vi "VIPM_Identify New and Modified Spec Files.vi"(7 "Force Reload?(F)":bool, 8 "error in (no error)":errorcluster, 11 "Spec Files":path[](array[path])) -> (0 "error out":errorcluster, 2 "New or Modified Spec Files":path[](array[path]), 3 "Unchanged Package Array":T1[](array[typedef]))   [LabVIEW 2019]
uses:
  Ctl/Ctl_Package Identifier Cluster.ctl
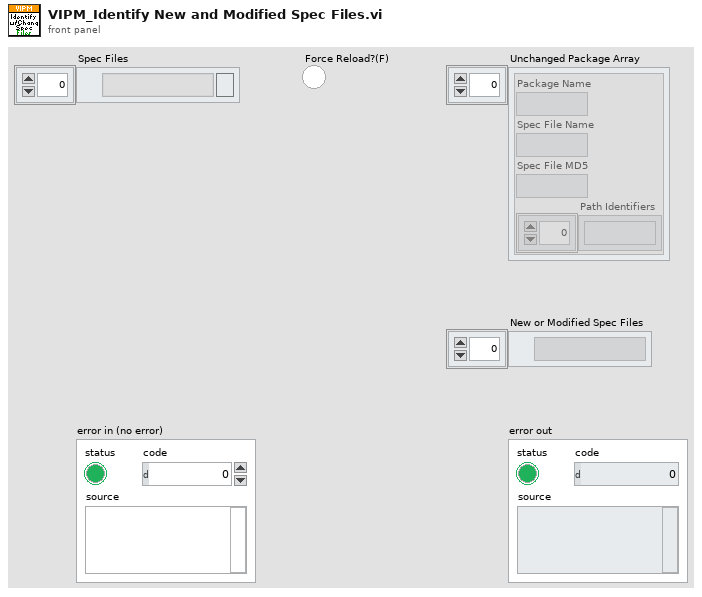
[diagram p1: front panel]
types:
  T1 = typedef "Ctl_Package Identifier Cluster.ctl" = cluster{"Package Name":string, "Spec File Name":string, "Spec File MD5":string, "Path Identifiers":string[]}
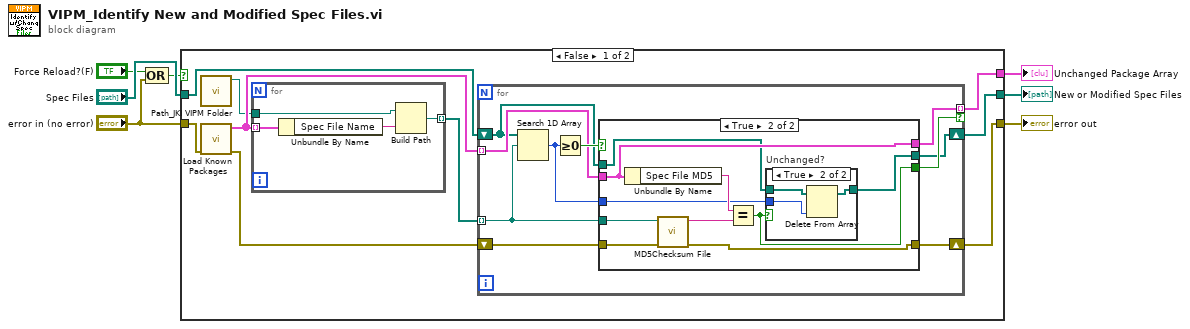
[diagram p0: block diagram]
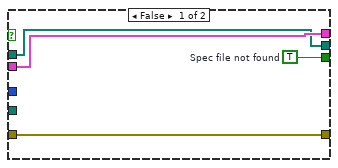
[diagram p2: hidden frame]
diagram:
  n1 = Compound Arithmetic op=OR("Force Reload?(F)", "error in (no error)") -> (w3:bool)
  n2 = case shown="False" w3 {
    tunnel: "Spec Files" -> [w13 w50]
    tunnel: [w12 _] -> w6
    tunnel: [w11 w50] -> w5
    tunnel: [w9 w49] -> w4
    tunnel: "error in (no error)" -> [w8 w49]
    frame False {
      n3 = call "Path_JKI VIPM Folder.vi"() -> ("JKI\\VIPM path"=w14:path)  [unwired: 10 in, 1 out]
      n4 = call "Load Known Packages.vi"("error in (no error)"=w8) -> ("error out"=w10:errorcluster, "Package Array from File"=w16:T1[])  [unwired: 8 in, 1 out]
      n5 = for {
        tunnel: w16 -> [w20] mode=indexing
        tunnel: [w17] -> w15 mode=indexing
        tunnel: w14 -> [w19]
        n6 = Unbundle By Name(w20) -> ("Spec File Name"=w18:string)
        n7 = Build Path(base path=w19, name or relative path=w18) -> (appended path=w17:path)
      }
      n8 = for {
        tunnel: w15 -> [w27] mode=indexing
        tunnel: w16 -> [w26] mode=indexing
        shift-right: [w23] -> w11
        shift-left: w13 -> [w24]
        tunnel: [w25] -> w12 mode=indexing if=w29
        shift-right: [w21] -> w9
        shift-left: w10 -> [w22]
        n9 = Search 1D Array(1D array=w24, element=w27) -> (index of element=w28:i32)  [unwired: 1 in]
        n10 = Greater Or Equal To 0?(x=w28) -> (x >= 0?=w30:bool)
        n11 = case shown="True" w30 {
          tunnel: [w34 w40] -> w29
          tunnel: w28 -> [_ w38]
          tunnel: w27 -> [_ w44]
          tunnel: w26 -> [w33 w41]
          tunnel: [w33 w41] -> w25
          tunnel: w24 -> [w32 w39]
          tunnel: [w32 w37] -> w23
          tunnel: w22 -> [w31 w36]
          tunnel: [w31 w35] -> w21
          frame False {
            w34 = TRUE  # Spec file not found
          }
          frame True {
            n12 = Unbundle By Name(w41) -> ("Spec File MD5"=w42:string)
            n13 = call <vilib>:"MD5Checksum File.vi"("error in (no error)"=w36, "Path"=w44) -> ("error out"=w35:errorcluster, "MD5 message-digest"=w43:string)  [unwired: 8 in]
            n14 = Equal?(x=w42, y=w43) -> (x = y?=w40:bool)
            n15 = case "Unchanged?" shown="True" w40 {
              tunnel: w39 -> [w45 w48]
              tunnel: w38 -> [_ w47]
              tunnel: [w45 w46] -> w37
              frame False {
              }
              frame True {
                n16 = Delete From Array(array=w48, index=w47) -> (array with subset deleted=w46:path[])  [unwired: 1 in, 1 out]
              }
            }
          }
        }
      }
    }
    frame True {
    }
  }
  "error out" <- w4
  "Unchanged Package Array" <- w6
  "New or Modified Spec Files" <- w5
